vi "StateSpaceUtil_IsDetectable.vi"(9 "C":T1, 11 "A":T1) -> (0 "Error":bool, 3 "IsDetectable":bool)   [LabVIEW 2019, in "Trajectory_Library.lvlib"]
doc: "Returns true if (A, B) is a stabilizable pair.\n \n(A,B) is stabilizable if and only if the uncontrollable eigenvalues of A, if any, have absolute values less than one, where an eigenvalue is uncontrollable if rank(?I - A, B) %3C n where n is number of states.\n \nInputs:\n - A -- System matrix.\n - B -- nput matrix.\n\nOutputs:\n - IsStablizable -- If the system is stabilizable."
uses:
  Trajectory_Library.lvlib
  <vilib>/Analysis/Matrix/Datatypes/RealMatrix.ctl
  <vilib>/Analysis/Matrix/NI_Matrix.lvlib
panel:
  # "<States, States>"
  # "<???, States>"
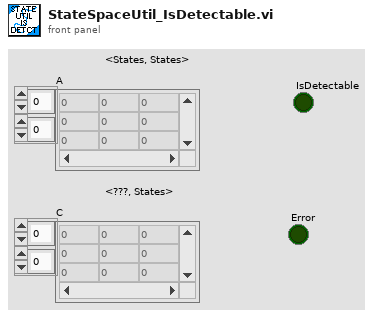
[diagram p1: front panel]
types:
  T1 = typedef "NI_Matrix.lvlib/RealMatrix.ctl" = dbl[][]
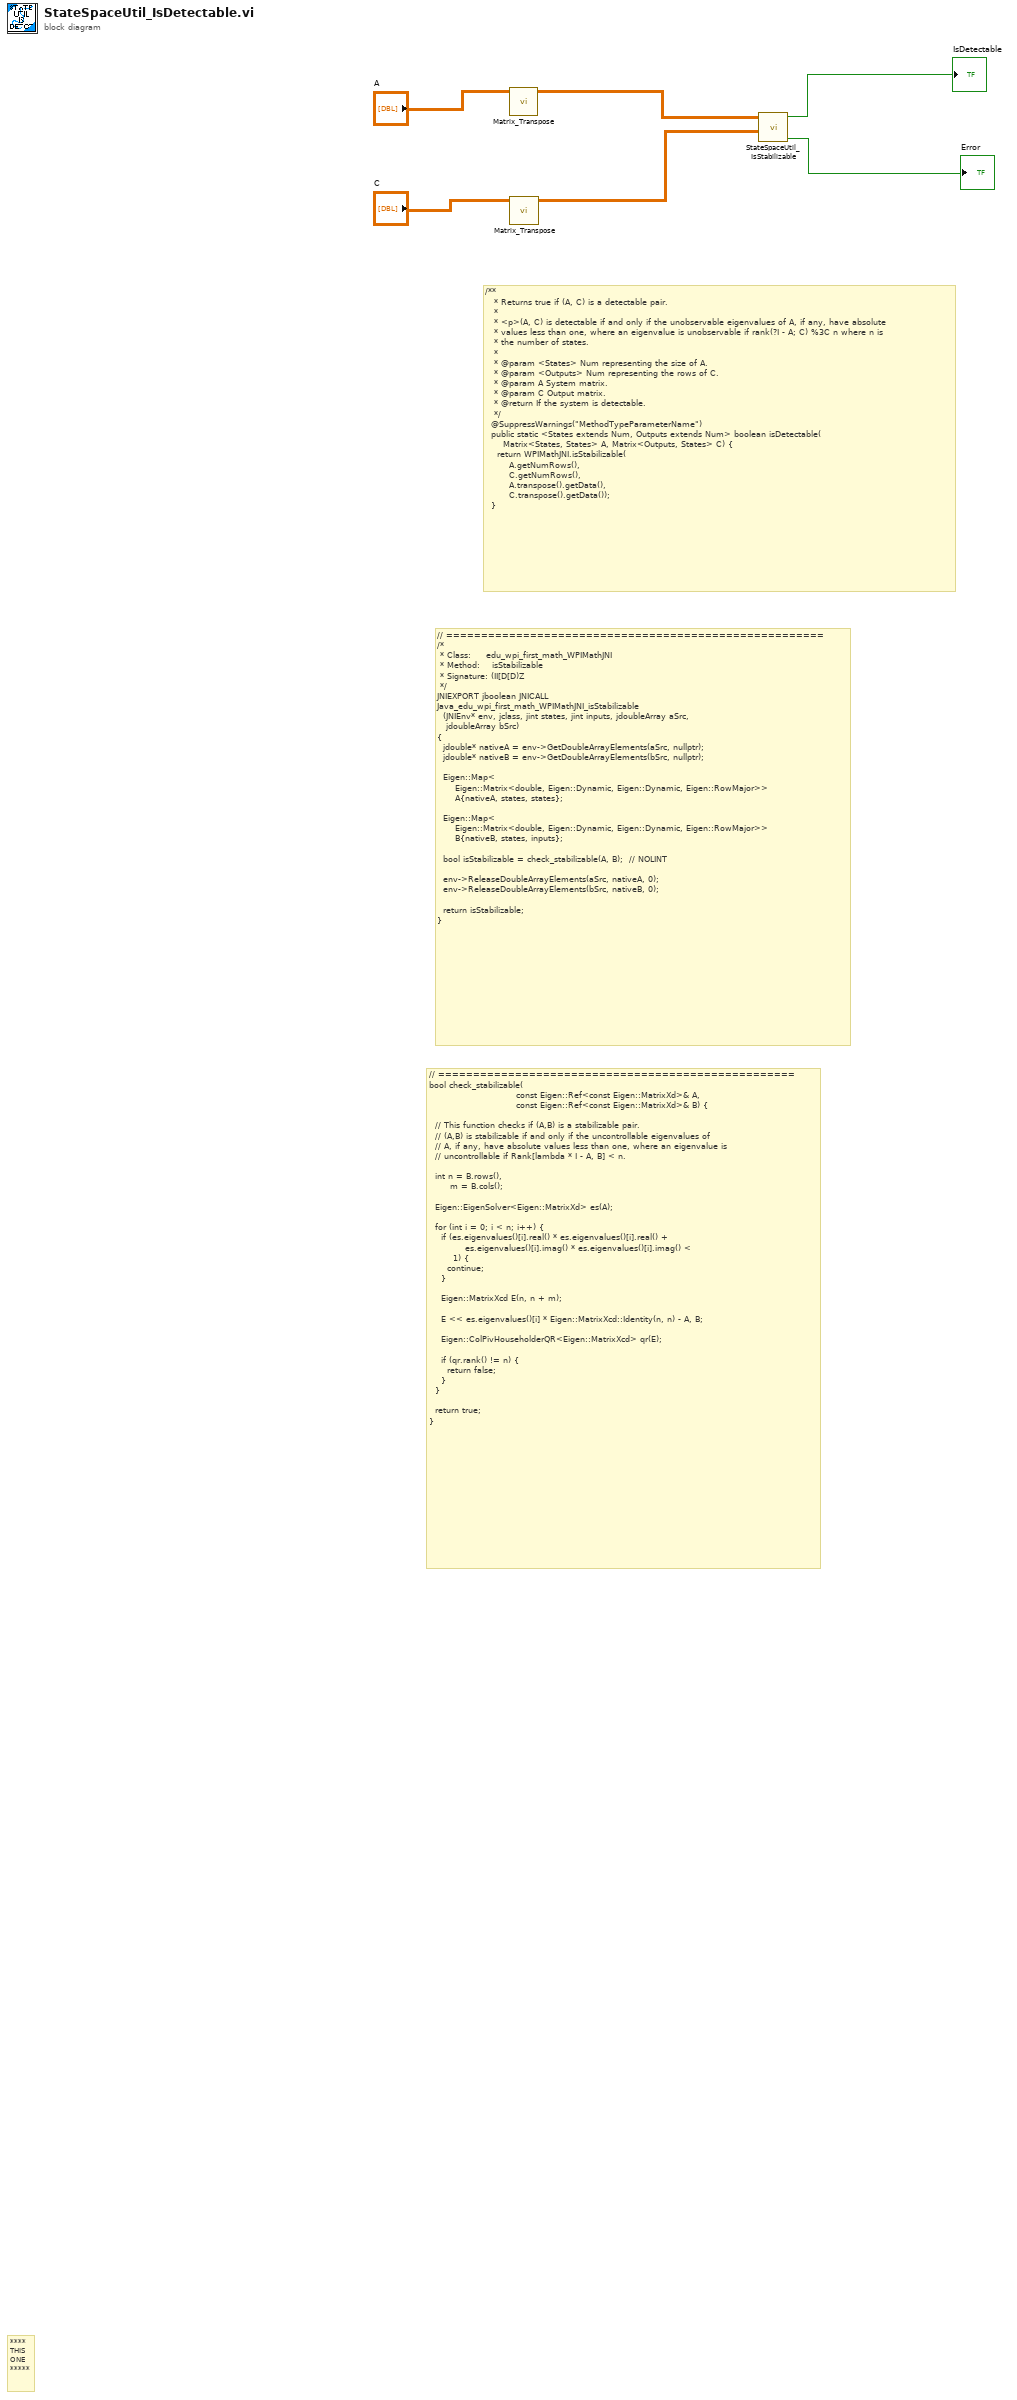
[diagram p0: block diagram]
diagram:
  # "/**\n   * Returns true if (A, C) is a detectable pair.\n   *\n   * <p>(A, C) is detectable if and only if the unobservable eigenvalues of A, if any, have absolute\n   * values less than one, where an eigenvalue is unobservable if rank(?I - A; C) %3C n where n is\n   * the number of states.\n   *\n   * @param <States> Num representing the size of A.\n   * @param <Outputs> Num representing the rows of C.\n   * @param A System matrix.\n   * @param C Output matrix.\n   * @return If the system is detectable.\n   */\n  @SuppressWarnings(\"MethodTypeParameterName\")\n  public static <States extends Num, Outputs extends Num> boolean isDetectable(\n      Matrix<States, States> A, Matrix<Outputs, States> C) {\n    return WPIMathJNI.isStabilizable(\n        A.getNumRows(), \n        C.getNumRows(), \n        A.transpose().getData(), \n        C.transpose().getData());\n  }"
  # "// ===================================================\nbool check_stabilizable(\n                             const Eigen::Ref<const Eigen::MatrixXd>& A,\n                             const Eigen::Ref<const Eigen::MatrixXd>& B) {\n\n  // This function checks if (A,B) is a stabilizable pair.\n  // (A,B) is stabilizable if and only if the uncontrollable eigenvalues of\n  // A, if any, have absolute values less than one, where an eigenvalue is\n  // uncontrollable if Rank[lambda * I - A, B] < n.\n\n  int n = B.rows(), \n       m = B.cols();\n\n  Eigen::EigenSolver<Eigen::MatrixXd> es(A);\n\n  for (int i = 0; i < n; i++) {\n    if (es.eigenvalues()[i].real() * es.eigenvalues()[i].real() +\n            es.eigenvalues()[i].imag() * es.eigenvalues()[i].imag() <\n        1) {\n      continue;\n    }\n\n    Eigen::MatrixXcd E(n, n + m);\n\n    E << es.eigenvalues()[i] * Eigen::MatrixXcd::Identity(n, n) - A, B;\n\n    Eigen::ColPivHouseholderQR<Eigen::MatrixXcd> qr(E);\n\n    if (qr.rank() != n) {\n      return false;\n    }\n  }\n\n  return true;\n}"
  # "// ======================================================\n/*\n * Class:     edu_wpi_first_math_WPIMathJNI\n * Method:    isStabilizable\n * Signature: (II[D[D)Z\n */\nJNIEXPORT jboolean JNICALL\nJava_edu_wpi_first_math_WPIMathJNI_isStabilizable\n  (JNIEnv* env, jclass, jint states, jint inputs, jdoubleArray aSrc,\n   jdoubleArray bSrc)\n{\n  jdouble* nativeA = env->GetDoubleArrayElements(aSrc, nullptr);\n  jdouble* nativeB = env->GetDoubleArrayElements(bSrc, nullptr);\n\n  Eigen::Map<\n      Eigen::Matrix<double, Eigen::Dynamic, Eigen::Dynamic, Eigen::RowMajor>>\n      A{nativeA, states, states};\n\n  Eigen::Map<\n      Eigen::Matrix<double, Eigen::Dynamic, Eigen::Dynamic, Eigen::RowMajor>>\n      B{nativeB, states, inputs};\n\n  bool isStabilizable = check_stabilizable(A, B);  // NOLINT\n\n  env->ReleaseDoubleArrayElements(aSrc, nativeA, 0);\n  env->ReleaseDoubleArrayElements(bSrc, nativeB, 0);\n\n  return isStabilizable;\n}"
  # "****\nTHIS\nONE\n*****"
  n1 = call "Matrix_Transpose.vi"("input matrix"="A") -> ("output matrix"=w4:T1)  [unwired: 10 in]
  n2 = call "Matrix_Transpose.vi"("input matrix"="C") -> ("output matrix"=w3:T1)  [unwired: 10 in]
  n3 = call "StateSpaceUtil_IsStabilizable.vi"("B"=w3, "A"=w4) -> ("Error"=→"Error":bool, "IsStabilizable"=→"IsDetectable":bool)  [unwired: 8 in]
